vi "ProjectVI.vi"() -> (3 "Max value of array":dbl, 11 "Sum of array":dbl)   [LabVIEW 2023]
doc: "Array = {5,3,9,8,1}\nOutput1 = Sum of array\nOutput2 = Max of array"
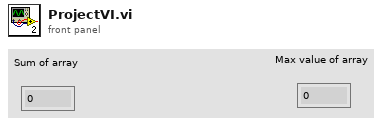
[diagram p1: front panel]
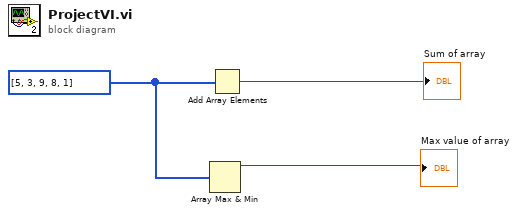
[diagram p0: block diagram]
diagram:
  w1 = i32[] [5, 3, 9, 8, 1]
  n1 = Array Max & Min(array=w1) -> (max value=→"Max value of array":i32)  [unwired: 3 out]
  n2 = Add Array Elements(numeric array=w1) -> (sum=→"Sum of array":i32)
